vi "Run Integration Tests.vi"(8 "Error In":errorcluster) -> (0 "Error Out":errorcluster)   [LabVIEW 2018, in "Scripts.lvlib"]
uses:
  Scripts.lvlib
  tests/Toolkit/Integration/Integration.lvlib
  <vilib>/addons/_JKI Toolkits/Caraya/classes/Test/Test.lvclass
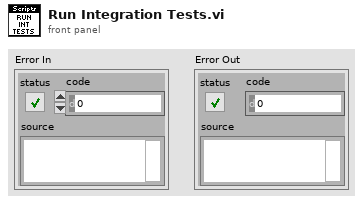
[diagram p1: front panel]
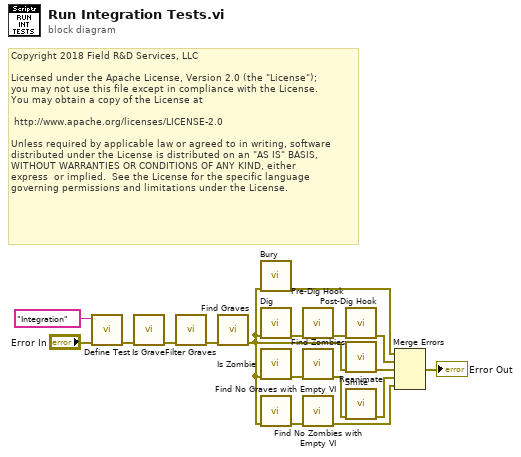
[diagram p0: block diagram]
diagram:
  # "Copyright 2018 Field R&D Services, LLC\n\nLicensed under the Apache License, Version 2.0 (the \"License\");\nyou may not use this file except in compliance with the License.\nYou may obtain a copy of the License at\n\n\thttp://www.apache.org/licenses/LICENSE-2.0\n\nUnless required by applicable law or agreed to in writing, software\ndistributed under the License is distributed on an \"AS IS\" BASIS,\nWITHOUT WARRANTIES OR CONDITIONS OF ANY KIND, either \nexpress  or implied.  See the License for the specific language \ngoverning permissions and limitations under the License."
  n1 = call <vilib>:"Define Test.vi"("error in (no error)"="Error In", "Label (VI Title)"="Integration") -> ("error out"=w11:errorcluster)  [unwired: 9 in]
  n2 = call "Is Grave.vi"("Error In"=w11) -> ("Error Out"=w13:errorcluster)  [unwired: 10 in]
  n3 = call "Filter Graves.vi"("Error In"=w13) -> ("Error Out"=w12:errorcluster)  [unwired: 10 in]
  n4 = call "Find Graves.vi"("Error In"=w12) -> ("Error Out"=w4:errorcluster)  [unwired: 10 in]
  n5 = call "Bury.vi"("Error In"=w4) -> ("Error Out"=w17:errorcluster)  [unwired: 10 in]
  n6 = call "Dig.vi"("Error In"=w4) -> ("Error Out"=w7:errorcluster)  [unwired: 10 in]
  n7 = call "Is Zombie.vi"("Error In"=w4) -> ("Error Out"=w14:errorcluster)  [unwired: 10 in]
  n8 = call "Find No Graves with Empty VI.vi"("Error In"=w4) -> ("Error Out"=w2:errorcluster)  [unwired: 10 in]
  n9 = call "Pre-Dig Hook.vi"("Error In"=w7) -> ("Error Out"=w6:errorcluster)  [unwired: 10 in]
  n10 = call "Find Zombies.vi"("Error In"=w14) -> ("Error Out"=w3:errorcluster)  [unwired: 10 in]
  n11 = call "Find No Zombies with Empty VI.vi"("Error In"=w2) -> ("Error Out"=w1:errorcluster)  [unwired: 10 in]
  n12 = call "Post-Dig Hook.vi"("Error In"=w6) -> ("Error Out"=w5:errorcluster)  [unwired: 10 in]
  n13 = call "Reanimate.vi"("Error In"=w4) -> ("Error Out"=w16:errorcluster)  [unwired: 10 in]
  n14 = call "Smite.vi"("Error In"=w3) -> ("Error Out"=w15:errorcluster)  [unwired: 10 in]
  n15 = Merge Errors(w17, w5, w16, w15, w1) -> (→"Error Out":errorcluster)
